vi "LV_ConTester.vi"() -> ()   [LabVIEW 2021]
uses:
  <vilib>/Instr/_visa.llb/VISA Configure Serial Port (Instr).vi
panel:
  in  "Tab Control":enum32{"Data", "Setup"}(tab)
  out "LED matrix":bool[][](array[boolean]) caption="Array"
  in  "Port":refnum<visa-resource-name>
  in  "baud rate (9600)":u32=9600
  in  "Bytes in packet":u32=24
  in  "?":bool
  out "Raw data":string
  out "Sync Error":bool
  out "CRC Error":bool
  # "INPUTS"
  # "1     2     3     4     5     6     7     8     9    10   11   12   13   14   15   16   17   18   19   20"
  # "1"
  # "2"
  # "3"
  # "4"
  # "OUTPUTS"
  # "5"
  # "6"
  # "7"
  # "8"
  # "COM Setup"
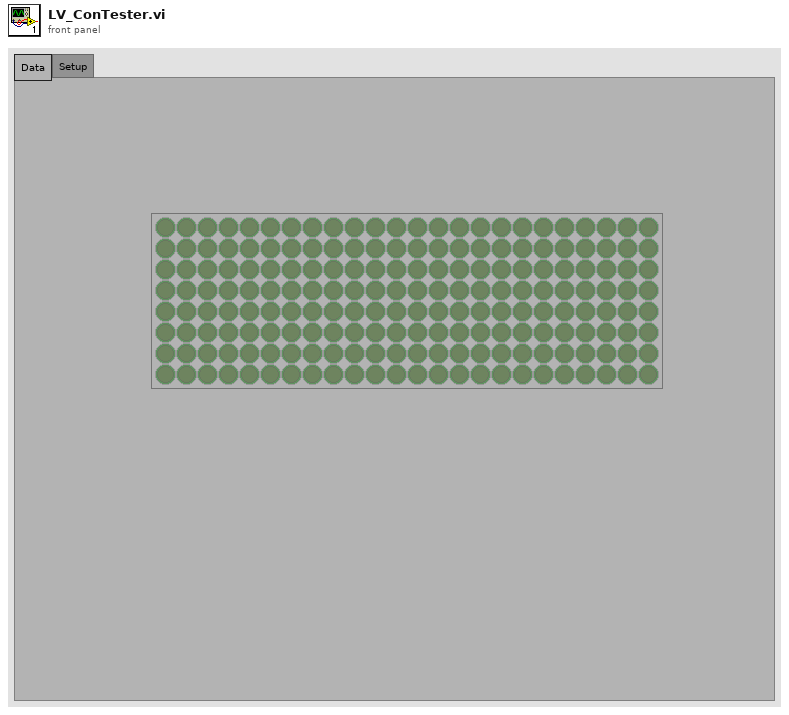
[diagram p1: front panel]
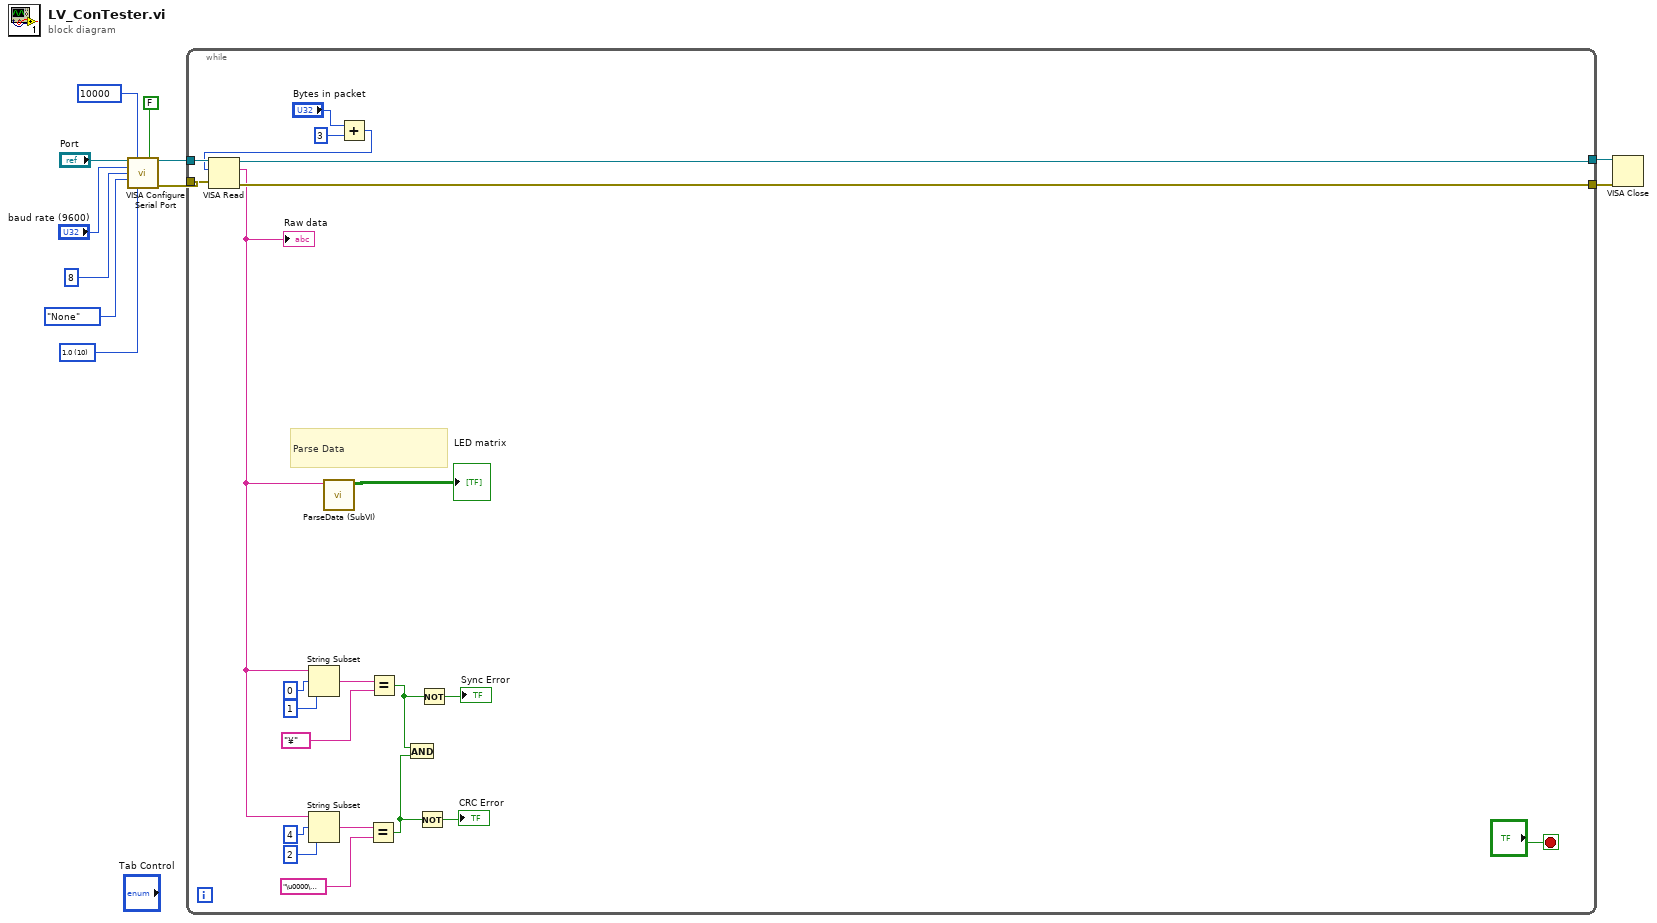
[diagram p0: block diagram]
diagram:
  w9 = u16 10 items=["1.0"=10, "1.5"=15, "2.0"=20] ("stop bits (10: 1 bit)")
  n1 = call-poly "VISA Configure Serial Port"("VISA resource name"="Port", "timeout (10sec)"=u32 10000, "Enable Termination\nChar (T)"=FALSE ("Enable Termination\nChar (T)"), "baud rate (9600)"="baud rate (9600)", "data bits (8)"=u16 8, "parity (0:none)"=enum16{"None", "Odd", "Even", "Mark", "Space"}."None", "stop bits (10: 1 bit)"=w9) -> ("VISA resource name out"=w3:refnum<visa-resource-name>, "error out"=w2:errorcluster)  [unwired: 7 in]
  n2 = while {
    tunnel: [w33] -> w11
    tunnel: [w32] -> w10
    tunnel: w3 -> [w31]
    tunnel: w2 -> [w30]
    stop <- "?" stop-if-true
    # "Parse Data"
    n3 = Add(x="Bytes in packet", y=u32 3) -> (x+y=w14:u32)
    n4 = VISA Read(VISA resource name=w31, byte count=w14, error in (no error)=w30) -> (VISA resource name out=w33:refnum<visa-resource-name>, read buffer=w13:string, error out=w32:errorcluster)  [unwired: 1 out]
    "Raw data" <- w13
    n5 = String Subset(string=w13, offset (0)=0, length (rest)=1 ("length (rest)")) -> (substring=w22:string)
    n6 = String Subset(string=w13, offset (0)=4, length (rest)=2 ("length (rest)")) -> (substring=w21:string)
    n7 = call "ParseData (SubVI).vi"("read buffer"=w13) -> ("Array"=→"LED matrix":bool[][])  [unwired: 10 in]
    n8 = Equal?(x=w21, y="\u0000\u0000") -> (x = y?=w17:bool)
    n9 = Equal?(x=w22, y="¥") -> (x = y?=w20:bool)
    n10 = And(x=w20, y=w17) -> ()  [unwired: 1 out]
    n11 = Not(x=w17) -> (.not. x?=→"CRC Error":bool)
    n12 = Not(x=w20) -> (.not. x?=→"Sync Error":bool)
  }
  n13 = VISA Close(VISA resource name=w11, error in (no error)=w10) -> ()  [unwired: 1 out]
